vi "CC WebRelay Get Status.vi"(8 "error in (no error)":errorcluster, 11 "connection ID":refnum<k5>) -> (0 "error out":errorcluster, 2 "status":bool[](array[boolean]), 3 "connection ID out":refnum<k5>)   [LabVIEW 2024]
uses:
  <vilib>/regexp/Match Regular Expression.xnode
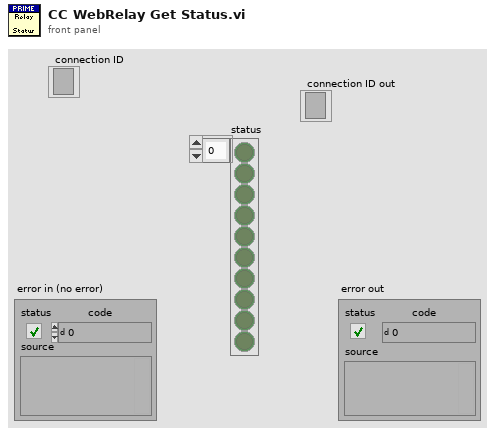
[diagram p1: front panel]
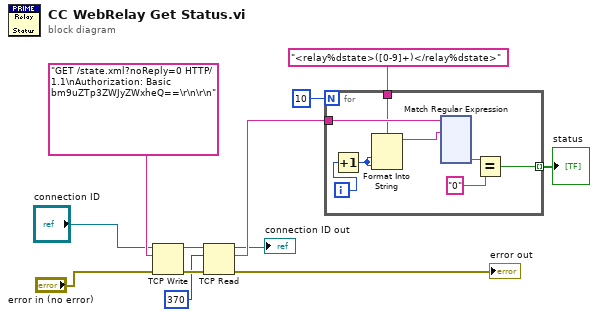
[diagram p0: block diagram]
diagram:
  n1 = TCP Write(connection ID="connection ID", data in="GET /state.xml?noReply=0 HTTP/1.1\nAuthorization: Basic bm9uZTp3ZWJyZWxheQ==\r\n\r\n", error in (no error)="error in (no error)") -> (connection ID out=w11:refnum<k5>, error out=w10:errorcluster)  [unwired: 1 in, 1 out]
  n2 = TCP Read(connection ID=w11, bytes to read=370, error in (no error)=w10) -> (connection ID out=→"connection ID out":refnum<k5>, data out=w7:string, error out=→"error out":errorcluster)  [unwired: 2 in]
  n3 = for {
    N: 10 -> [_]
    tunnel: w7 -> [w20]
    tunnel: "<relay%dstate>([0-9]+)</relay%dstate>" ("regular expression") -> [w19]
    tunnel: [w13] -> w1 mode=indexing
    i -> [w18]
    n4 = Increment(x=w18) -> (x+1=w16:i32)
    n5 = Format Into String(format string=w19, w16, w16) -> (resulting string=w17:string)  [unwired: 2 in, 1 out]
    n6 = xnode "Match Regular Expression"("input string"=w20, "regular expression"=w17) -> ("submatch 1"=w15:string)  [unwired: 4 in, 5 out]
    n7 = Equal?(x=w15, y="0") -> (x = y?=w13:bool)
  }
  "status" <- w1
